vi "RP hub read.vi"(4 "timeout ms (25000)":i32=250000, 6 "Bytes per sample":i32=4, 8 "Error In":errorcluster, 9 "hub port":u64=2, 10 "Number of samples":u64, 11 "connection ID":refnum<k5>) -> (0 "Error Out":errorcluster, 2 "data out":string, 3 "connection ID out":refnum<k5>)   [LabVIEW 2024]
uses:
  RP Command.ctl
  RP Write Command TCP.vi
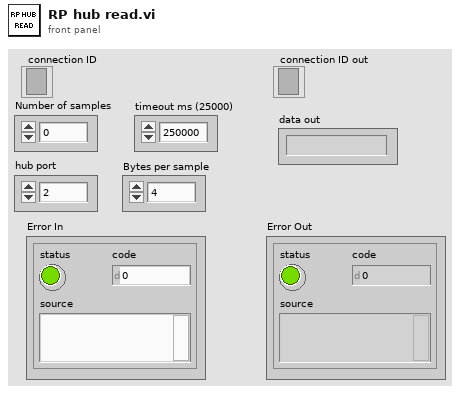
[diagram p1: front panel]
types:
  T1 = typedef "RP Command.ctl" = enum16{"Reset", "Read IDN", "Stop server", "Get status", "Get temperature", "Connect client", "Arm", "Software trigger", "Get whole buffer", "Get chunk", "System call", "Get config", "Set config", "Recieve data", "Recieve Calibartion", "Transmit data"}
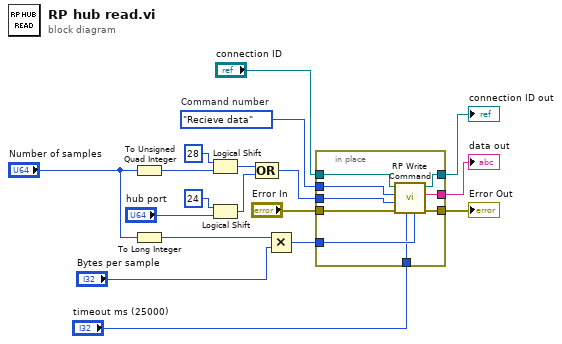
[diagram p0: block diagram]
diagram:
  w14 = RP_Command."Recieve data"  # Command number
  n1 = To Unsigned Quad Integer(1:"Number of samples") -> (0:w8:u64)
  n2 = To Long Integer(number="Number of samples") -> (32bit integer=w3:i32)
  n3 = Logical Shift(y=i16 28, x=w8) -> (x << y=w10:u64)
  n4 = Logical Shift(y=i16 24, x="hub port") -> (x << y=w9:u64)
  n5 = Compound Arithmetic op=OR(w10, w9) -> (w7:u64)
  n6 = Multiply(x=w3, y="Bytes per sample") -> (x*y=w4:i32)
  n7 = in-place {
    in-place-border: "connection ID" -> [w27]
    in-place-border: [w21] -> w17
    in-place-border: [w22] -> w16
    in-place-border: "Error In" -> [w26]
    in-place-border: w14 -> [w25]
    in-place-border: w7 -> [w24]
    in-place-border: w4 -> [w23]
    in-place-border: [w20] -> w2
    in-place-border: "timeout ms (25000)" -> [w19]
    n8 = call-poly "RP Write Command.vi"("bytes to read"=w23, "timeout ms (25000)"=w19, "Error In"=w26, "Command payload"=w24, "Command number"=w25, "connection ID"=w27) -> ("Error Out"=w21:errorcluster, "data out"=w20:string, "connection ID out"=w22:refnum<k5>)  [unwired: 2 in, 1 out]
  }
  "connection ID out" <- w16
  "Error Out" <- w17
  "data out" <- w2
